vi "Depth_Controller_run.vi"(8 "error in (no error)":errorcluster) -> (0 "error out":errorcluster)   [LabVIEW 2013]
uses:
  My Computer/Controls/EKF_Settings.ctl
  My Computer/Controls/SpaceMouse_Buttons.ctl
  My Computer/Controls/Estimated Position.ctl
  My Computer/Controls/Swimbladder Tuning Parameters.ctl
  My Computer/Controls/Advanced Swimbladder Indicators.ctl
panel:
  out "Duty Cycle [-]":dbl
  out "Motor Current [A]":dbl
  out "Duty cycle before":dbl
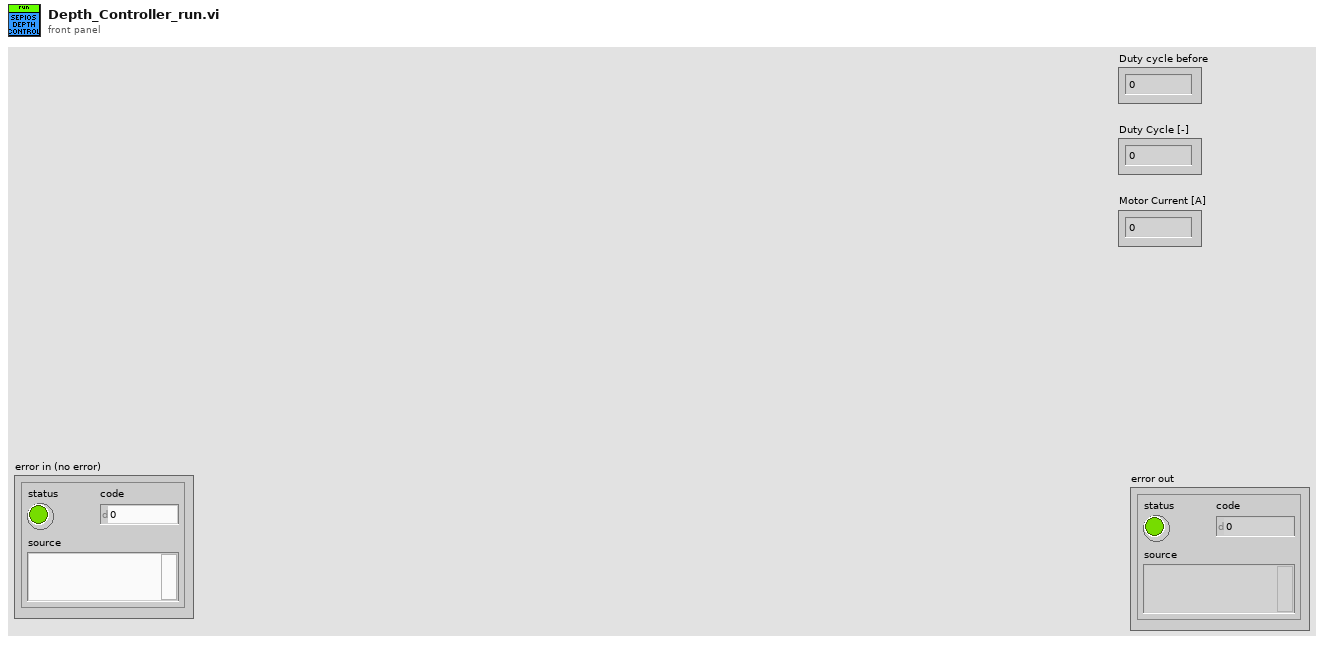
[diagram p1: front panel]
types:
  T1 = typedef "EKF_Settings.ctl" = cluster{"Gravity constant":dbl, "Filter Version":enum16{"IMU Only", "IMU & Pressure", "IMU, Pressure, Compass"}, "Initial Biases":cluster{"Gyro_Bias_nit_x":dbl, "Gyro_Bias_init_y":dbl, "Gyro_Bias_init_z":dbl, "Acc_Bias_init_x":dbl, "Acc_Bias_init_y":dbl, "Acc_Bias_init_z":dbl}, "Use Compass on initialisation":bool, "Initial Biases Covariances":cluster{"Initial_covariance_Gyro_Bias":dbl, "Initial_covariance_Acc_Bias":dbl}, "Magnetic-Field-Vector [utesla]":cluster{"Magf_N_x":dbl, "Magf_N_y":dbl, "Magf_N_z":dbl}, "IMU_Sigmas":cluster{"Sigma_w":dbl, "Sigma_wb":dbl, "Sigma_a":dbl, "Sigma_ab":dbl, "Sigma_m":dbl}, "Measurement Sigmas":cluster{"Sigma_v":dbl, "Sigma_depth":dbl}}
  T2 = enum16{"IMU Only", "IMU & Pressure", "IMU, Pressure, Compass"}
  T3 = typedef "SpaceMouse_Buttons.ctl" = cluster{"Idle":bool, "Button Right":bool, "Button Left":bool}
  T4 = typedef "Estimated Position.ctl" = cluster{"X":dbl, "Y":dbl, "Z":dbl, "V_X":dbl, "V_Y":dbl, "V_Z":dbl}
  T5 = typedef "Swimbladder Tuning Parameters.ctl" = cluster{"Excessive_Depth_Deviation_Trigger":dbl, "Neutral Buoancy_x":dbl, "Ti_Depth_Control":dbl, "kp_Depth_Control":dbl, "Integrator enabled range Depth":dbl, "Integrator_enable_Range_Motor":dbl, "kp_Motor":dbl, "Ti_Motor":dbl}
  T6 = typedef "Advanced Swimbladder Indicators.ctl" = cluster{"P_ref [Pa]":dbl, "X_Actual [m]":dbl, "Motor Current[A]":dbl}
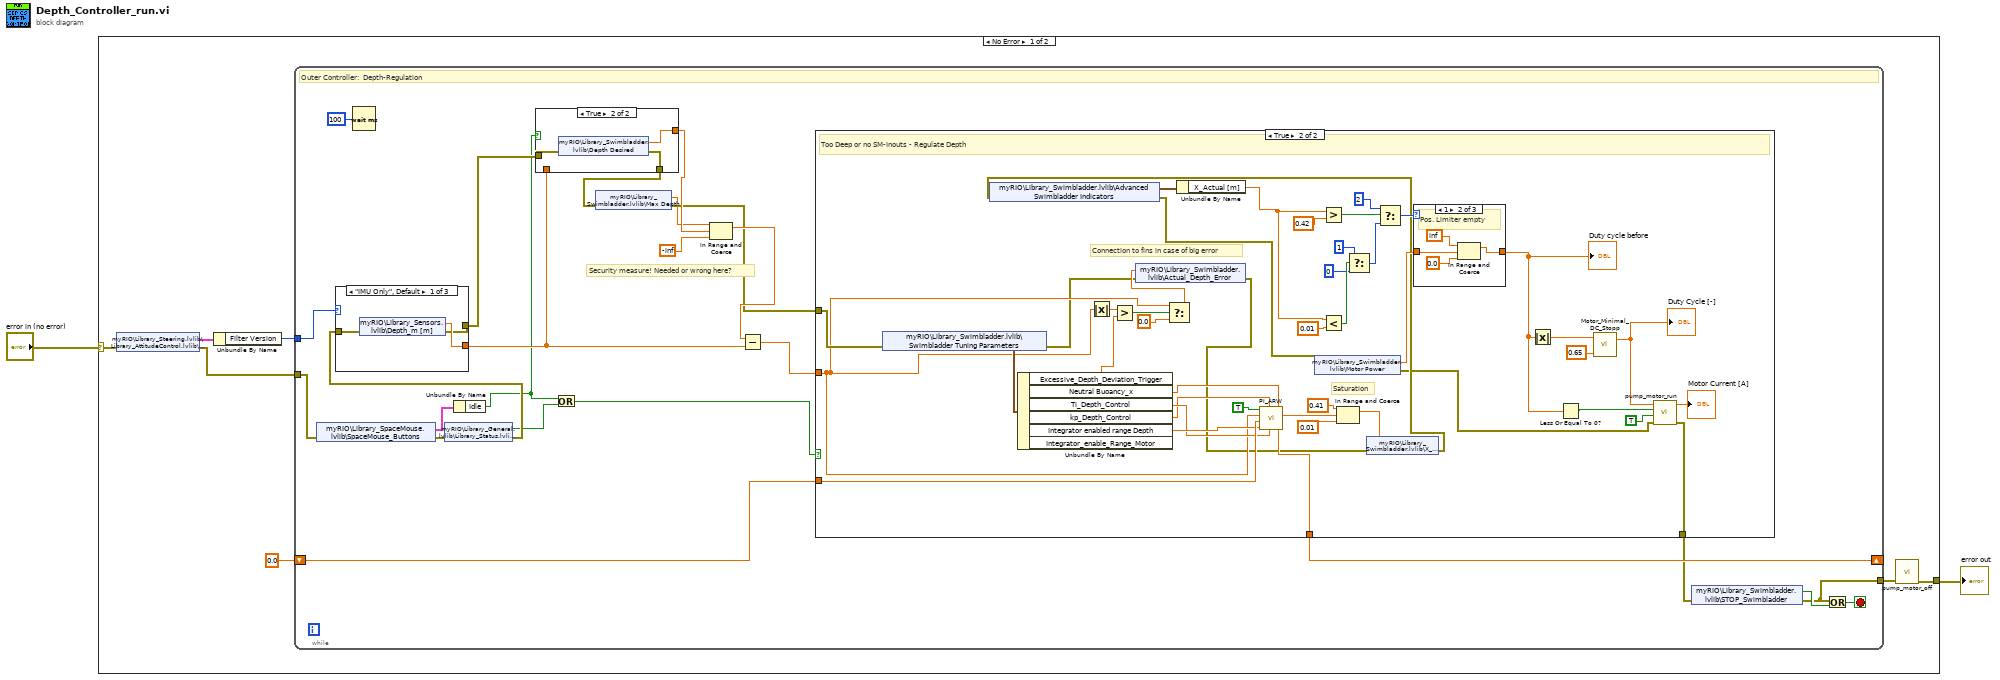
[diagram p0: block diagram]
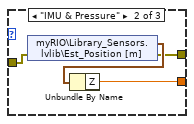
[diagram p2: hidden frame]
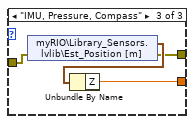
[diagram p3: hidden frame]
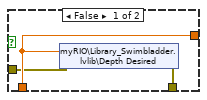
[diagram p4: hidden frame]
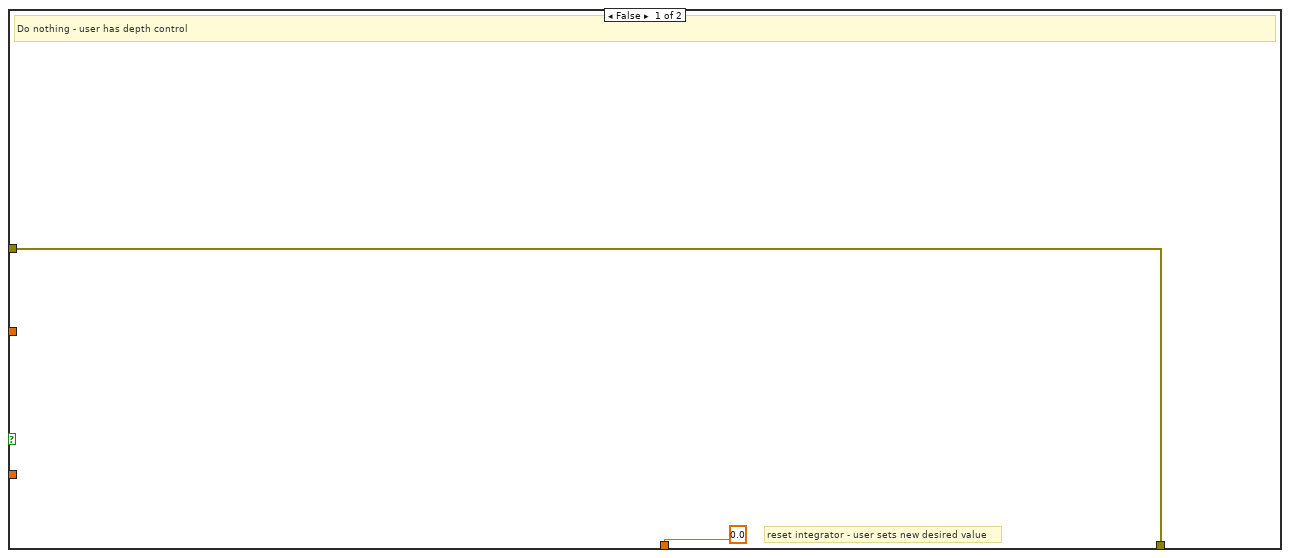
[diagram p5: hidden frame]
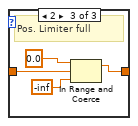
[diagram p7: hidden frame]
diagram:
  n1 = case shown="No Error" "error in (no error)" {
    selector: "error in (no error)" -> [w5 w106]
    tunnel: [w7 w106] -> w2
    frame No Error {
      n2 = shared-variable "myRIO\\Library_Steering.lvlib\\Library_AttitudeControl.lvlib\\EKF_Settings"(error in=w5) -> (w6:T1, error out=w4:errorcluster)
      n3 = Unbundle By Name(w6) -> ("Filter Version"=w3:T2)
      n4 = while {
        tunnel: w4 -> [w22]
        tunnel: [w31] -> w8
        shift-right: [w30] -> _
        shift-left: 0.0 -> [w29]
        tunnel: w3 -> [w18]
        stop <- w33 stop-if-true
        # "Security measure! Needed or wrong here?"
        # "Outer Controller:  Depth-Regulation"
        n5 = shared-variable "myRIO\\Library_SpaceMouse.lvlib\\SpaceMouse_Buttons"(error in=w22) -> (w23:T3, error out=w21:errorcluster)
        n6 = Wait (ms)(milliseconds to wait=u32 100) -> ()  [unwired: 1 out]
        n7 = shared-variable "myRIO\\Library_General.lvlib\\Library_Status.lvlib\\tooDeep"(error in=w21) -> (w12:bool, error out=w17:errorcluster)
        n8 = case shown="\"IMU Only\", Default" w18 {
          tunnel: [w35 w39 w43] -> w15
          tunnel: w17 -> [w36 w38 w42]
          tunnel: [w34 w37 w41] -> w16
          frame "IMU Only", Default {
            n9 = shared-variable "myRIO\\Library_Sensors.lvlib\\Depth_m [m]"(error in=w36) -> (w35:dbl, error out=w34:errorcluster)
          }
          frame "IMU & Pressure" {
            n10 = shared-variable "myRIO\\Library_Sensors.lvlib\\Est_Position [m]"(error in=w38) -> (w40:T4, error out=w37:errorcluster)
            n11 = Unbundle By Name(w40) -> ("Z"=w39:dbl)
          }
          frame "IMU, Pressure, Compass" {
            n12 = shared-variable "myRIO\\Library_Sensors.lvlib\\Est_Position [m]"(error in=w42) -> (w44:T4, error out=w41:errorcluster)
            n13 = Unbundle By Name(w44) -> ("Z"=w43:dbl)
          }
        }
        n14 = Unbundle By Name(w23) -> ("Idle"=w13:bool)
        n15 = case shown="True" w13 {
          tunnel: [w46 w50] -> w27
          tunnel: w16 -> [w45 w49]
          tunnel: [w47 w48] -> w20
          tunnel: w15 -> [w46 _]
          frame False {
            n16 = shared-variable "myRIO\\Library_Swimbladder.lvlib\\Depth Desired"(w46, error in=w45) -> (error out=w47:errorcluster)
          }
          frame True {
            n17 = shared-variable "myRIO\\Library_Swimbladder.lvlib\\Depth Desired"(error in=w49) -> (w50:dbl, error out=w48:errorcluster)
          }
        }
        n18 = Or(x=w13, y=w12) -> (x .or. y?=w24:bool)
        n19 = shared-variable "myRIO\\Library_Swimbladder.lvlib\\Max Depth"(error in=w20) -> (w11:dbl, error out=w14:errorcluster)
        n20 = In Range and Coerce(upper limit=w11, x=w27, lower limit=-inf) -> (coerced(x)=w28:dbl)  [unwired: 1 out]
        n21 = Subtract(x=w28, y=w15) -> (x-y=w26:dbl)
        n22 = case shown="True" w24 {
          tunnel: [w52 w95] -> w25
          tunnel: [0.0 ("new error") w77] -> w30
          tunnel: w29 -> [_ w76]
          tunnel: w14 -> [w52 w72]
          tunnel: w26 -> [_ w64]
          frame False {
            # "reset integrator - user sets new desired value"
            # "Do nothing - user has depth control"
          }
          frame True {
            # "Connection to fins in case of big error"
            # "Saturation"
            # "Too Deep or no SM-Inouts - Regulate Depth"
            n23 = shared-variable "myRIO\\Library_Swimbladder.lvlib\\Swimbladder Tuning Parameters"(error in=w72) -> (w73:T5, error out=w56:errorcluster)
            n24 = Unbundle By Name(w73) -> ("Excessive_Depth_Deviation_Trigger"=w71:dbl, "Neutral Buoancy_x"=w68:dbl, "Ti_Depth_Control"=w69:dbl, "kp_Depth_Control"=w57:dbl, "Integrator enabled range Depth"=w70:dbl)  [unwired: 1 out]
            n25 = Absolute Value(x=w64) -> (abs(x)=w74:dbl)
            n26 = Greater?(x=w74, y=w71) -> (0:w65:bool)
            n27 = Select(t=w64, s=w65, f=0.0) -> (s? t:f=w62:dbl)
            n28 = shared-variable "myRIO\\Library_Swimbladder.lvlib\\Actual_Depth_Error"(w62, error in=w56) -> (error out=w55:errorcluster)
            n29 = call "PI_ARW.vi"("offset"=w68, "Ti_value"=w69, "p_value"=w57, "Integrator enabled range"=w70, "old error"=w76, "actual error"=w64, "ARW on/off"=TRUE) -> ("new error"=w77:dbl, "output"=w78:dbl)  [unwired: 1 in]
            n30 = In Range and Coerce(upper limit=0.41, x=w78, lower limit=0.01) -> (coerced(x)=w58:dbl)  [unwired: 1 out]
            n31 = shared-variable "myRIO\\Library_Swimbladder.lvlib\\X_desired"(w58, error in=w55) -> (error out=w54:errorcluster)
            n32 = shared-variable "myRIO\\Library_Swimbladder.lvlib\\Advanced Swimbladder Indicators"(error in=w54) -> (w59:T6, error out=w60:errorcluster)
            n33 = Unbundle By Name(w59) -> ("X_Actual [m]"=w61:dbl)
            n34 = shared-variable "myRIO\\Library_Swimbladder.lvlib\\Motor Power"(error in=w60) -> (w87:dbl, error out=w53:errorcluster)
            n35 = Greater?(x=w61, y=0.42) -> (0:w86:bool)
            n36 = Less?(x=w61, y=0.01) -> (x < y?=w85:bool)
            n37 = Select(t=1, s=w85, f=0) -> (s? t:f=w81:i32)
            n38 = Select(t=2, s=w86, f=w81) -> (s? t:f=w80:i32)
            n39 = case shown="1" w80 {
              tunnel: w87 -> [w97 w100 w105]
              tunnel: [w97 w99 w104] -> w67
              frame 0, Default {
                # "Pos. Limiter normal"
              }
              frame 1 {
                # "Pos. Limiter empty"
                n40 = In Range and Coerce(upper limit=inf, x=w100, lower limit=0.0) -> (coerced(x)=w99:dbl)  [unwired: 1 out]
              }
              frame 2 {
                # "Pos. Limiter full"
                n41 = In Range and Coerce(upper limit=0.0, x=w105, lower limit=-inf) -> (coerced(x)=w104:dbl)  [unwired: 1 out]
              }
            }
            "Duty cycle before" <- w67
            n42 = Absolute Value(x=w67) -> (abs(x)=w92:dbl)
            n43 = Less Or Equal To 0?(x=w67) -> (x <= 0?=w66:bool)
            n44 = call "Motor_Minimal_DC_Stopp.vi"("Turn_off_Trigger_Duty-Cylce"=0.65, "Desired Duty-Cycle"=w92) -> ("Triggered Duty-Cycle"=w93:dbl)  [unwired: 2 in]
            "Duty Cycle [-]" <- w93
            n45 = call "pump_motor_run.vi"("error in (no error)"=w53, "Enable"=TRUE, "Empty Swim Bladder"=w66, "PWM Duty Cycle [0, 1]"=w93) -> ("error out"=w95:errorcluster, "Motor Current[A]"=→"Motor Current [A]":dbl)  [unwired: 5 in, 1 out]
          }
        }
        n46 = shared-variable "myRIO\\Library_Swimbladder.lvlib\\STOP_Swimbladder"(error in=w25) -> (w32:bool, error out=w31:errorcluster)
        n47 = Or(x=w31, y=w32) -> (x .or. y?=w33:bool)
      }
      n48 = call "pump_motor_off.vi"("error in (no error)"=w8) -> ("error out"=w7:errorcluster)  [unwired: 10 in]
    }
    frame Error {
    }
  }
  "error out" <- w2
